vi "Write ctl.vi"(8 "error in (no error)":errorcluster, 10 "ctl":cluster{"p":dbl, "i":dbl, "d":dbl}, 11 "TEC in":refnum<class "TEC.lvclass">) -> (0 "error out":errorcluster, 3 "TEC out":refnum<class "TEC.lvclass">)   [LabVIEW 2014, in "Generic TEC.lvlib" / "TEC.lvclass"]
uses:
  TEC.lvclass
  TEC.lvclass/TEC.ctl
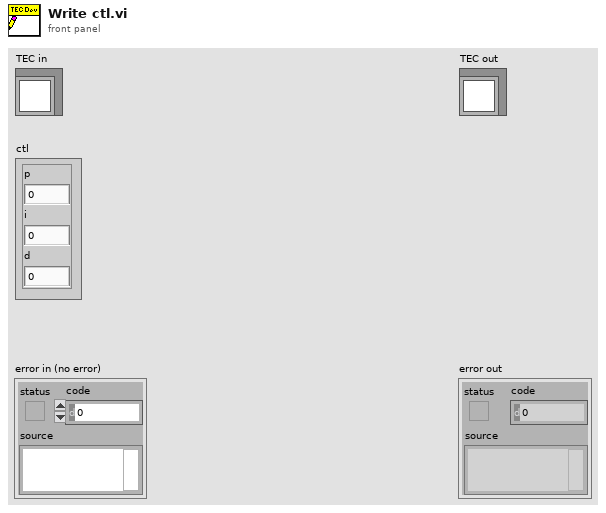
[diagram p1: front panel]
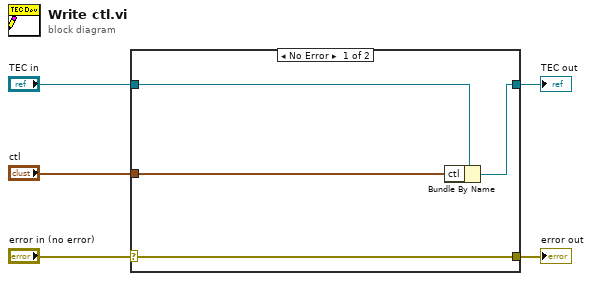
[diagram p0: block diagram]
diagram:
  n1 = case shown="No Error" "error in (no error)" {
    selector: "error in (no error)" -> [w9 w10]
    tunnel: [w9 w10] -> w4
    tunnel: [w7 w11] -> w2
    tunnel: "TEC in" -> [w8 w11]
    tunnel: "ctl" -> [w6 _]
    frame No Error {
      n2 = Bundle By Name(cluster=w8, "ctl"=w6) -> (w7:refnum<class "TEC.lvclass">)
    }
    frame Error {
    }
  }
  "error out" <- w4
  "TEC out" <- w2
